vi "CreateIntegerArray.vi"(8 "Spacing":enum16{"Linear", "Logrithmic"}(ring), 9 "# of Points":i32, 10 "Maximum":i32, 11 "Minimum":i32) -> (3 "Array":i32[](array[numeric]))   [LabVIEW 2014]
uses:
  <vilib>/imath/engines/lvmath2/RunTimeEngine/BuiltInFunctions/linramp/NIMS_linramp.vi
  <vilib>/imath/engines/lvmath2/RunTimeEngine/NodeEndStatement/NIMS_NodeEndStatement_Output.vi
  <instcachedir>/0/NIMS_NodeEndStatement_Output_53EC0D466D134D7ABD903AC30B43404B.lvgen/NIMS_NodeEndStatement_Output_53EC0D466D134D7ABD903AC30B43404B_004.vi
  <vilib>/imath/engines/lvmath2/RunTimeEngine/ErrorHandling/NIMS_Finalize Error.vi
  <vilib>/imath/engines/lvmath2/RunTimeSupport/NIMS_Complex To Real.vi
  <instcachedir>/0/NIMS_Complex To Real_CFEFC05793354143908F7AF8F5FCAA9D.lvgen/NIMS_Complex To Real_CFEFC05793354143908F7AF8F5FCAA9D_001.vi
  <vilib>/imath/engines/lvmath2/RunTimeEngine/BuiltInFunctions/logramp/NIMS_logramp.vi
  <vilib>/imath/engines/lvmath2/RunTimeEngine/ErrorHandling/NIMS_Create Error From Enums.vi
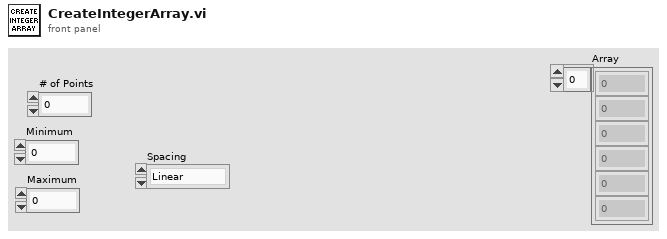
[diagram p1: front panel]
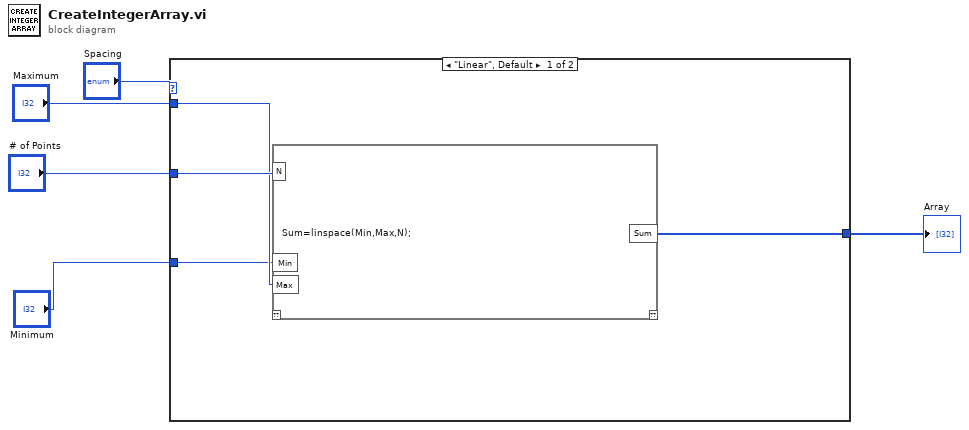
[diagram p0: block diagram]
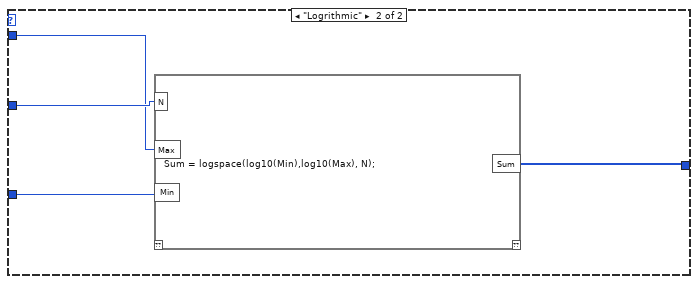
[diagram p2: hidden frame]
diagram:
  n1 = case shown="\"Linear\", Default" "Spacing" {
    tunnel: "# of Points" -> [w9 w39]
    tunnel: "Maximum" -> [w8 w37]
    tunnel: "Minimum" -> [w7 w38]
    tunnel: [w6 w36] -> w2
    frame "Linear", Default {
      n2 = mathscript code="Sum=linspace(Min,Max,N);"("N"=w9, "Min"=w7, "Max"=w8) -> ("Sum"=w6:i32[])  [unwired: 1 in, 1 out]
    }
    frame "Logrithmic" {
      n3 = mathscript code="Sum = logspace(log10(Min),log10(Max), N);"("N"=w39, "Min"=w38, "Max"=w37) -> ("Sum"=w36:i32[])  [unwired: 1 in, 1 out]
    }
  }
  "Array" <- w2
